vi "HMSET.vi"(0 "refnum in":refnum<vi>, 1 "Key":string, 5 "Fields":string[](array[string]), 7 "Values":string[](array[string]), 11 "error in":errorcluster) -> (4 "refnum out":refnum<vi>, 6 "Data":T1, 15 "error out":errorcluster)   [LabVIEW 2020]
uses:
  SubVIs/Controls/redis-data.ctl
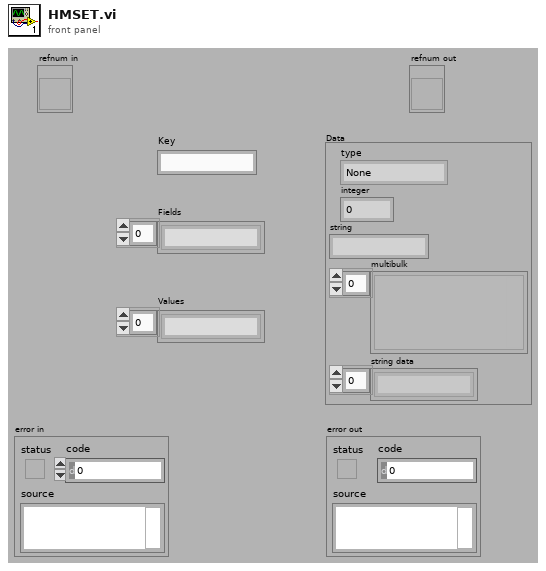
[diagram p1: front panel]
types:
  T1 = typedef "redis-data.ctl" = cluster{"type":enum16{"None", "Error", "Status", "Nil", "Integer", "String", "Multibulk"}, "integer":i64, "string":string, "multibulk":variant[], "string data":string[]}
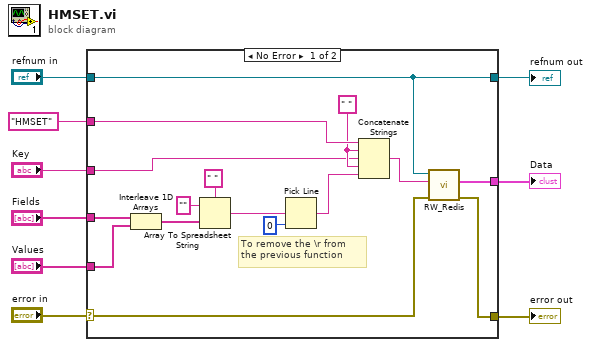
[diagram p0: block diagram]
diagram:
  n1 = case shown="No Error" "error in" {
    selector: "error in" -> [w19 w27]
    tunnel: "Fields" -> [w14 _]
    tunnel: "HMSET" -> [w12 _]
    tunnel: "refnum in" -> [w16 w26]
    tunnel: [w18 w27] -> w5
    tunnel: [w17 _] -> w4
    tunnel: [w16 w26] -> w3
    tunnel: "Values" -> [w15 _]
    tunnel: "Key" -> [w10 _]
    frame No Error {
      w11 = " "
      # "To remove the \\r from\nthe previous function"
      n2 = Interleave 1D Arrays(w14, w15) -> (w13:string[])
      n3 = Array To Spreadsheet String(delimiter (Tab)=" ", array=w13, 3:"" ("format string")) -> (spreadsheet string=w22:string)
      n4 = Pick Line(multi-line string=w22, line index=0) -> (output string=w23:string)  [unwired: 1 in]
      n5 = Concatenate Strings(w12, w11, w10, w11, w23) -> (w20:string)
      n6 = call "RW_Redis.vi"("error in"=w19, "command"=w20, "refnum"=w16) -> ("error out"=w18:errorcluster, "Data"=w17:T1)  [unwired: 7 in]
    }
    frame Error {
    }
  }
  "error out" <- w5
  "Data" <- w4
  "refnum out" <- w3
